vi "useexternaldep.vi"() -> ()   [LabVIEW 2017]
uses:
  includes/PPL.lvlibp
panel:
  out "Numeric 2":dbl
  in  "Numeric":dbl
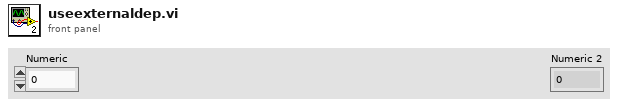
[diagram p1: front panel]
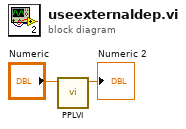
[diagram p0: block diagram]
diagram:
  n1 = call "PPLVI.vi"("Numeric"="Numeric") -> ("Numeric 2"=→"Numeric 2":dbl)  [unwired: 10 in]
